vi "Set DAQmxTask_.vi"(8 "error in (no error)":errorcluster, 9 "DAQmxTask":refnum<class "DAQmxTask.lvclass">, 10 "Task name":string, 11 "DAQmxTaksContainer_General in":refnum<class "DAQmxTaksContainer_General.lvclass">) -> (0 "error out":errorcluster, 3 "DAQmxTaksContainer_General out":refnum<class "DAQmxTaksContainer_General.lvclass">)   [LabVIEW 2015, in "DAQmxTaksContainer_General.lvclass"]
uses:
  DAQmxTaksContainer_General.lvclass
  DAQmxTask.lvclass
  DAQmxTaksContainer_General.lvclass/DAQmxTaksContainer_General.ctl
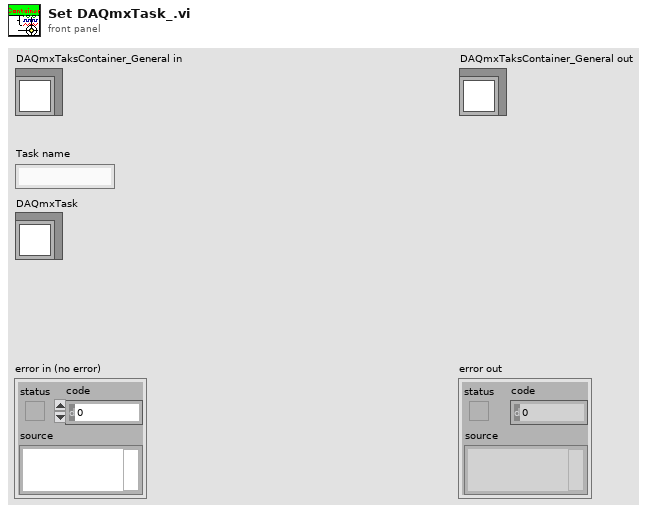
[diagram p1: front panel]
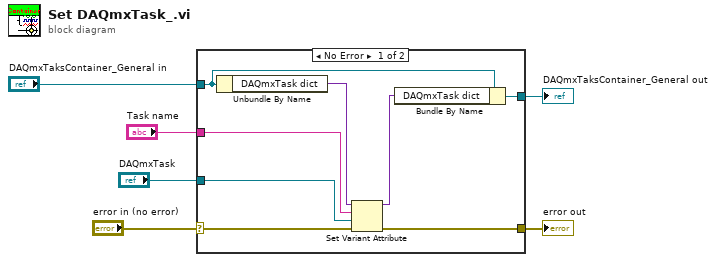
[diagram p0: block diagram]
diagram:
  n1 = case shown="No Error" "error in (no error)" {
    selector: "error in (no error)" -> [w11 w16]
    tunnel: [w10 w16] -> w3
    tunnel: [w8 w15] -> w2
    tunnel: "DAQmxTaksContainer_General in" -> [w9 w15]
    tunnel: "Task name" -> [w13 _]
    tunnel: "DAQmxTask" -> [w12 _]
    frame No Error {
      n2 = Unbundle By Name(w9) -> ("DAQmxTask dict"=w14:variant)
      n3 = Set Variant Attribute(Variant=w14, name=w13, value=w12, error in=w11) -> (Variant out=w7:variant, error out=w10:errorcluster)  [unwired: 1 out]
      n4 = Bundle By Name(cluster=w9, "DAQmxTask dict"=w7) -> (w8:refnum<class "DAQmxTaksContainer_General.lvclass">)
    }
    frame Error {
    }
  }
  "error out" <- w3
  "DAQmxTaksContainer_General out" <- w2
